vi "Item Ref to BaseNodeType.vi"(8 "error in (no error)":errorcluster, 11 "Item Ref":u64) -> (0 "error out":errorcluster, 3 "BaseNodeType":refnum<k24>)   [LabVIEW 2017, in "SLSC Switch Import Unit Tests.lvclass"]
uses:
  SLSC Switch Import Unit Tests.lvclass
  NationalInstruments.VeriStand.SystemStorage
  NationalInstruments.VeriStand.SystemDefinitionAPI
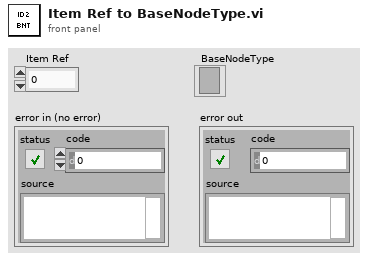
[diagram p1: front panel]
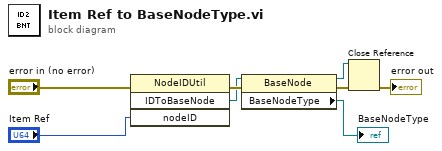
[diagram p0: block diagram]
diagram:
  n1 = invoke class="NodeIDUtil" method="IDToBaseNode"(error in="error in (no error)", "nodeID"="Item Ref") -> (error out=w5:errorcluster, "IDToBaseNode"=w4:refnum<k24>)  [unwired: 2 in, 2 out]
  n2 = property class="BaseNode"(reference=w4, error in=w5) -> (reference out=w1:refnum<k24>, error out=w7:errorcluster, "BaseNodeType"=→"BaseNodeType":refnum<k24>)
  n3 = Close Reference(reference=w1, error in (no error)=w7) -> (error out=→"error out":errorcluster)
